vi "Led Color.vi"() -> ()   [LabVIEW 2020]
uses:
  <vilib>/nisyscfg/nisyscfg.lvlib
  <resource>/objmgr/nicriosae.rc
  <resource>/objmgr/nisysapi.rc
  <vilib>/nisyscfg/Close (Hardware).vi
  <vilib>/nisyscfg/Close (System).vi
  <vilib>/nisyscfg/Close (Filter).vi
  <vilib>/nisyscfg/Save Changes (Hardware).vi
panel:
  out "Devices & Chassis:Model Name Number":u32
  out "Simulated?":bool
  in  "Led Status":u32(ring) items=["Off"=0, "Solid Green"=1, "Solid Yellow"=2, "Blinking Green"=4, "Blinking Yellow"=8]
  in  "Device Name":string
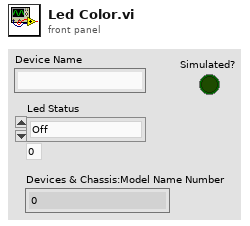
[diagram p1: front panel]
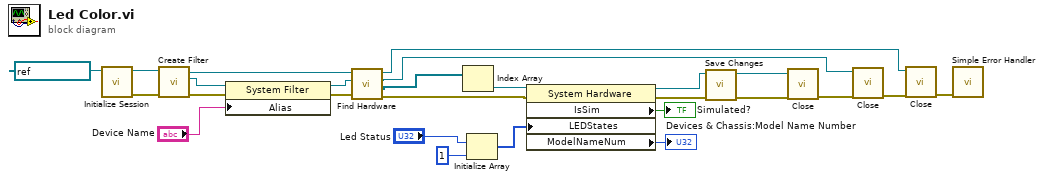
[diagram p0: block diagram]
diagram:
  n1 = call <vilib>:"Initialize Session.vi"("Target (localhost)"=refnum<k21> "localhost" ("Device Name")) -> ("error out"=w21:errorcluster, "Session out"=w22:refnum<k21>)  [unwired: 9 in]
  n2 = call <vilib>:"Create Filter.vi"("error in (no error)"=w21, "Session in"=w22) -> ("error out"=w26:errorcluster, "Filter out"=w25:refnum<k20>, "Session out"=w23:refnum<k21>)  [unwired: 7 in]
  n3 = property class="System Filter"(reference=w25, error in=w26, "Alias"="Device Name") -> (reference out=w1:refnum<k20>, error out=w24:errorcluster)
  n4 = call <vilib>:"Find Hardware.vi"("error in (no error)"=w24, "Filter in"=w1, "Session in"=w23) -> ("error out"=w15:errorcluster, "Resources out"=w20:refnum<k20>[], "Filter out"=w17:refnum<k20>, "Session out"=w10:refnum<k21>)  [unwired: 5 in]
  n5 = Index Array(array=w20) -> (element=w16:refnum<k20>)  [unwired: 1 in]
  n6 = Initialize Array("Led Status", 1 ("dimension size")) -> (w5:u32[])
  n7 = property class="System Hardware"(reference=w16, error in=w15, "LEDStates"=w5) -> (reference out=w13:refnum<k20>, error out=w12:errorcluster, "IsSim"=→"Simulated?":bool, "ModelNameNum"=→"Devices & Chassis:Model Name Number":u32)
  n8 = call-poly <vilib>:"Save Changes.vi"("error in (no error)"=w12, "Resource in"=w13) -> ("error out"=w8:errorcluster, "Resource out"=w11:refnum<k20>)  [unwired: 6 in, 2 out]
  n9 = call-poly <vilib>:"Close.vi"("error in (no error)"=w8, "Resource in"=w11) -> ("error out"=w18:errorcluster)  [unwired: 9 in]
  n10 = call-poly <vilib>:"Close.vi"("error in (no error)"=w18, "Filter in"=w17) -> ("error out"=w19:errorcluster)  [unwired: 9 in]
  n11 = call-poly <vilib>:"Close.vi"("error in (no error)"=w19, "Session in"=w10) -> ("error out"=w9:errorcluster)  [unwired: 9 in]
  n12 = call <vilib>:"Simple Error Handler.vi"("error in (no error)"=w9) -> ()  [unwired: 4 in, 5 out]
